vi "Cache.vi"(11 "Idx":i32) -> ()   [LabVIEW 2016]
uses:
  Cache.Data.ctl
  Cache.Data.Status.ctl
  Cache.Data.Sets.ctl
  Cache.Action.ctl
  Tools/CitTemplate/citTemplate.errData.ctl
  Tools/EventLog/EventLog.EventSource.ctl
  Database/Database.Global.vi
panel:
  out "error.action":string
  out "error":errorcluster
  out "_loop":i32(ring)=4
  out "action":T1=enum."--- Cache ---"
  out "Data":T2
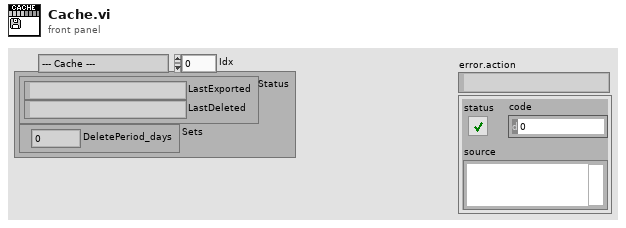
[diagram p1: front panel]
types:
  T1 = typedef "Cache.Action.ctl" = enum32{"idle", "constructor", "destructor", "--- Cache ---", "Find", "FindToExport", "Move", "Delete"}
  T2 = typedef "Cache.Data.ctl" = cluster{"Status":T3, "Sets":T4}
  T3 = typedef "Cache.Data.Status.ctl" = cluster{"LastExported":string, "LastDeleted":string}
  T4 = typedef "Cache.Data.Sets.ctl" = cluster{"DeletePeriod_days":dbl}
  T5 = typedef "citTemplate.errData.ctl" = cluster{"ts":timestamp, "src":T6, "instance":i32, "action":string, "error":errorcluster, "unconfirmed":bool}
  T6 = typedef "EventLog.EventSource.ctl" = enum16{"All", "Gui", "Cache", "PLC1", "PLC2", "PLC3", "DB", "DB01", "DB02", "DB03", "DB04", "DB05", "DB06", "DB07", "DB08", "DB09", "DB10", "DB11", "DB12", "DB13", "DB14", "DB15", "DB16"}
  T7 = cluster{"File":path, "Time (now)":timestamp, "error in":errorcluster}
  T8 = typedef "citTemplate.notifierHandle.ctl" = refnum<notifier>
  T9 = typedef "ProdaNG.ProductComponent.ctl" = cluster{"product_wabcoNumber":string, "product_serialNumber":string, "component_wabcoNumber":string, "component_serialNumber":string, "pressStepResultId":string, "qty":i32, "level":i32}
  T10 = typedef "Cache.TestSteps.Fglb.ResultData.ctl" = cluster{"File":path, "Ref":string, "Serial":string, "Pr":T11, "PSr":T12, "TSr":cluster{"TSr":T13, "TVr":T14[]}[]}
  T11 = typedef "ProdaNG.ProcessResult.ctl" = cluster{"c_id":string, "productId":string, "processId":i32, "statusId":i32, "startTime":string, "endTime":string}
  T12 = typedef "ProdaNG.ProcessStepResult.ctl" = cluster{"c_id":string, "processResultId":string, "processStepId":i32, "statusId":i32, "operatorId":i32, "startTime":string, "endTime":string}
  T13 = typedef "ProdaNG.TestStepResult.ctl" = cluster{"c_id":string, "processStepResultId":string, "testStepId":i32, "statusId":i32}
  T14 = typedef "ProdaNG.TestValueResult.ctl" = cluster{"c_id":string, "testStepResultId":string, "testValueId":i32, "result":dbl, "statusId":i32, "contentId":string}
  T15 = cluster{"Results":T10[], "ProductComponent":T9[]}
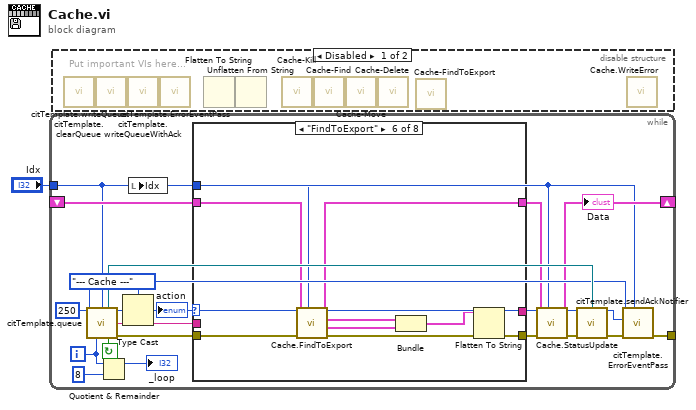
[diagram p0: block diagram]
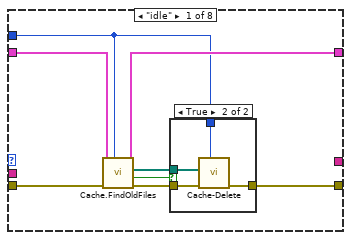
[diagram p3: hidden frame]
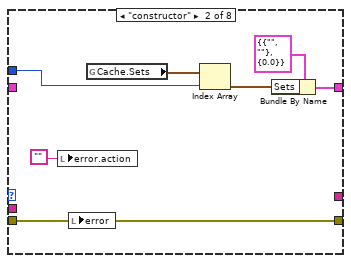
[diagram p5: hidden frame]
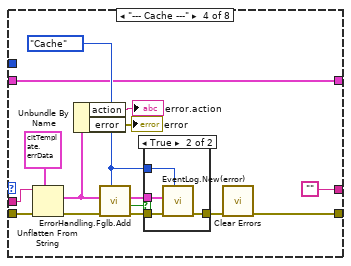
[diagram p7: hidden frame]
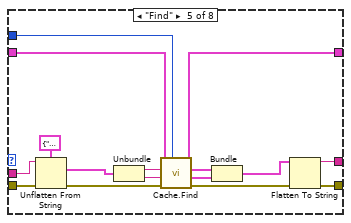
[diagram p9: hidden frame]
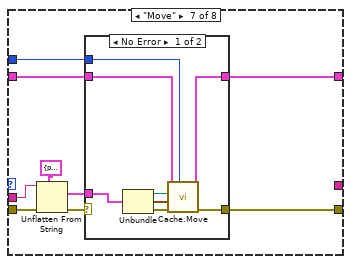
[diagram p10: hidden frame]
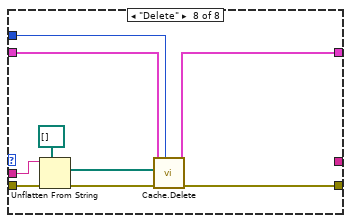
[diagram p12: hidden frame]
diagram:
  n1 = while {
    tunnel: [w14] -> _
    shift-right: [w3] -> _
    shift-left: _ -> [w7]
    tunnel: "Idx" -> [w2]
    i -> [w15]
    stop <- w17 continue-if-true
    w8 = Cache.Action."--- Cache ---" ("Action")
    n2 = call "citTemplate.queue.vi"("ms timeout (250 ms)"=250, "instance (0)"=w2, "event enum"=w8, "iteration (-1)"=w15) -> ("notifierHandle out"=w9:T8, "event out"=w20:u32, "(flatten) data out"=w19:string, "continue"=w17:bool, "error out"=w18:errorcluster)  [unwired: 1 in, 6 out]
    n3 = Quotient & Remainder(x=w15, y=8) -> (x-y*floor(x/y)=→"_loop":i32)  [unwired: 1 out]
    n4 = Type Cast(type=w8, x=w20) -> (*(type *) &x=w13:T1)
    "action" <- w13
    n5 = local write "Idx"(w2) -> ()
    n6 = case shown="\"FindToExport\"" w13 {
      tunnel: w19 -> [_ _ _ w54 w68 _ w95 w110]
      tunnel: w18 -> [w28 w39 w41 w56 w69 w79 w96 w111]
      tunnel: [w24 w39 w41 w45 w71 w81 w89 w112] -> w6
      tunnel: [w26 w34 w42 w43 w75 w85 w92 w114] -> w4
      tunnel: w7 -> [w27 _ w42 w43 w76 w86 w93 w115]
      tunnel: [_ _ _ "" w70 w80 _ _] -> w10
      tunnel: w2 -> [w21 w36 _ _ w77 w87 w94 w113]
      frame "idle" {
        n7 = call "Cache.FindOldFiles.vi"("Idx"=w21, "error in"=w28, "Data in"=w27) -> ("error out"=w25:errorcluster, "Found?"=w22:bool, "files to remove"=w23:path[], "Data out"=w26:T2)  [unwired: 5 in]
        n8 = case shown="True" w22 {
          tunnel: w25 -> [w29 w33]
          tunnel: [w29 w32] -> w24
          tunnel: w23 -> [_ w31]
          tunnel: w21 -> [_ w30]
          frame False {
          }
          frame True {
            n9 = call "Cache-Delete.vi"("Idx"=w30, "error in"=w33, "Files"=w31) -> ("error out"=w32:errorcluster)  [unwired: 8 in]
          }
        }
      }
      frame "constructor" {
        n10 = local write "error.action"("" ("error.action")) -> ()
        n11 = local write "error"(w39) -> ()
        n12 = global read "Database.Global.vi" "Cache.Sets"() -> (w38:T4[])
        n13 = Index Array(array=w38, index=w36) -> (element=w37:T4)
        n14 = Bundle By Name(cluster=T2 {"Status"={"LastExported"="", "LastDeleted"=""}, "Sets"={"DeletePeriod_days"=0.0}} ("Data"), "Sets"=w37) -> (w34:T2)
      }
      frame "destructor" {
      }
      frame "--- Cache ---" {
        w46 = EventLog.EventSource."Cache" ("Event source")
        n15 = Unflatten From String(type=T5 {"ts"=timestamp(0 s since 1904-01-01), "src"=enum."All", "instance"=0, "action"="", "error"={"status"=FALSE, "code"=0, "source"=""}, "unconfirmed"=FALSE} ("ErrData"), binary string=w54, error in (no error)=w56) -> (value=w48:T5, error out=w50:errorcluster)  [unwired: 3 out]
        n16 = Unbundle By Name(w48) -> ("action"=→"error.action":string, "error"=→"error":errorcluster)
        n17 = call "ErrorHandling.Fglb.Add.vi"("Event source"=w46, "error in (no error)"=w50, "Error in"=w48) -> ("error out"=w52:errorcluster, "changed?"=w51:bool)  [unwired: 7 in]
        n18 = case shown="True" w51 {
          tunnel: [w57 w61] -> w49
          tunnel: w48 -> [_ w60]
          tunnel: w52 -> [w57 w59]
          tunnel: w46 -> [_ w58]
          frame False {
          }
          frame True {
            n19 = call "EventLog.New(error).vi"("Source (All)"=w58, "error in"=w59, "ErrData"=w60) -> ("error out"=w61:errorcluster)  [unwired: 8 in]
          }
        }
        n20 = call <vilib>:"Clear Errors.vi"("error in (no error)"=w49) -> ("error out"=w45:errorcluster)  [unwired: 5 in, 1 out]
      }
      frame "Find" {
        n21 = Unflatten From String(type=cluster{"Variant":string, "Serial":string} {"Variant"="", "Serial"=""} ("cluster"), binary string=w68, error in (no error)=w69) -> (value=w66:cluster{"Variant":string, "Serial":string}, error out=w63:errorcluster)  [unwired: 2 in, 1 out]
        n22 = Unbundle(w66) -> ("Variant"=w64:string, "Serial"=w65:string)
        n23 = call "Cache.Find.vi"("Idx"=w77, "error in (no error)"=w63, "Serial"=w65, "Variant"=w64, "Data in"=w76) -> ("error out"=w74:errorcluster, "ProductComponent"=w72:T9, "Result"=w73:T10, "Data out"=w75:T2)  [unwired: 3 in]
        n24 = Bundle("Result"=w73, "ProductComponent"=w72) -> (w62:cluster{"Result":T10, "ProductComponent":T9})  [unwired: 1 in]
        n25 = Flatten To String(anything=w62, error in (no error)=w74) -> (data string=w70:string, error out=w71:errorcluster)  [unwired: 2 in, 1 out]
      }
      frame "FindToExport" {
        n26 = call "Cache.FindToExport.vi"("Idx"=w87, "error in (no error)"=w79, "Data in"=w86) -> ("error out"=w84:errorcluster, "ProductComponent"=w82:T9[], "Results"=w83:T10[], "Data out"=w85:T2)  [unwired: 5 in]
        n27 = Bundle("Results"=w83, "ProductComponent"=w82) -> (w78:T15)  [unwired: 1 in]
        n28 = Flatten To String(anything=w78, error in (no error)=w84) -> (data string=w80:string, error out=w81:errorcluster)  [unwired: 2 in, 1 out]
      }
      frame "Move" {
        n29 = Unflatten From String(type=T7 {"File"=path "", "Time (now)"=timestamp(0 s since 1904-01-01), "error in"={"status"=FALSE, "code"=0, "source"=""}} ("cluster"), binary string=w95, error in (no error)=w96) -> (value=w90:T7, error out=w88:errorcluster)  [unwired: 2 in, 1 out]
        n30 = case shown="No Error" w88 {
          selector: w88 -> [_ w106]
          tunnel: w94 -> [w104 _]
          tunnel: w93 -> [w103 w105]
          tunnel: [w102 w105] -> w92
          tunnel: w90 -> [w97 _]
          tunnel: [w98 w106] -> w89
          frame No Error {
            n31 = Unbundle(w97) -> ("File"=w101:path, "Time (now)"=w100:timestamp, "error in"=w99:errorcluster)
            n32 = call "Cache.Move.vi"("Idx"=w104, "error in"=w99, "Time (now)"=w100, "file"=w101, "Data in"=w103) -> ("error out"=w98:errorcluster, "Data out"=w102:T2)  [unwired: 5 in]
          }
          frame Error {
          }
        }
      }
      frame "Delete" {
        n33 = Unflatten From String(type=path[] [] ("files to remove"), binary string=w110, error in (no error)=w111) -> (value=w107:path[], error out=w108:errorcluster)  [unwired: 2 in, 1 out]
        n34 = call "Cache.Delete.vi"("Idx"=w113, "error in"=w108, "Files"=w107, "Data in"=w115) -> ("error out"=w112:errorcluster, "Data out"=w114:T2)  [unwired: 6 in]
      }
    }
    n35 = call "Cache.StatusUpdate.vi"("Idx"=w2, "error in (no error)"=w6, "Data in"=w4) -> ("error out"=w5:errorcluster, "Data out"=w3:T2)  [unwired: 7 in]
    "Data" <- w3
    n36 = call "citTemplate.sendAckNotifier.vi"("notification data"=w10, "notifierHandle in"=w9, "error in"=w5) -> ()  [unwired: 13 in]
    n37 = call "citTemplate.ErrorEventPass.vi"("instance"=w2, "error in"=w5, "action of error"=w13, "event in"=w8) -> ("error out"=w14:errorcluster)  [unwired: 1 in, 6 out]
  }
  n38 = disable-structure shown="Disabled" {
    frame Disabled {
      # "Put important VIs here..."
      n39 = call "citTemplate.clearQueue.vi"() -> ()  [unwired: 14 in, 2 out]
      n40 = call "citTemplate.writeQueue.vi"() -> ()  [unwired: 15 in, 1 out]
      n41 = call "citTemplate.writeQueueWithAck.vi"() -> ()  [unwired: 13 in, 3 out]
      n42 = call "citTemplate.ErrorEventPass.vi"() -> ()  [unwired: 11 in, 1 out]
      n43 = Flatten To String() -> ()  [unwired: 4 in, 3 out]
      n44 = Unflatten From String() -> ()  [unwired: 5 in, 3 out]
      n45 = call "Cache-Kill.vi"() -> ()  [unwired: 11 in, 1 out]
      n46 = call "Cache-Find.vi"() -> ()  [unwired: 8 in, 4 out]
      n47 = call "Cache-Move.vi"() -> ()  [unwired: 11 in, 1 out]
      n48 = call "Cache-Delete.vi"() -> ()  [unwired: 11 in, 1 out]
      n49 = call "Cache-FindToExport.vi"() -> ()  [unwired: 9 in, 3 out]
      n50 = call "Cache.WriteError.vi"() -> ()  [unwired: 10 in, 2 out]
    }
    frame Enabled {
    }
  }
